vi "FiltJump.vi"(9 "LowLim":sgl, 10 "HighLim":sgl, 11 "Path":T2) -> (3 "PathOut":T2)   [LabVIEW 2014]
uses:
  TypeDefs/Point2DwSlope.ctl
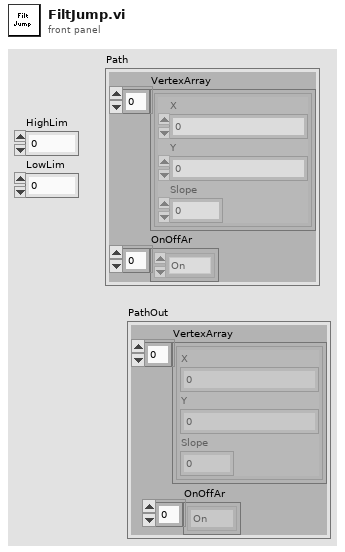
[diagram p1: front panel]
types:
  T1 = typedef "Point2DwSlope.ctl" = cluster{"X":sgl, "Y":sgl, "Slope":dbl}
  T2 = cluster{"VertexArray":T1[], "OnOffAr":enum16{"On", "Off"}[]}
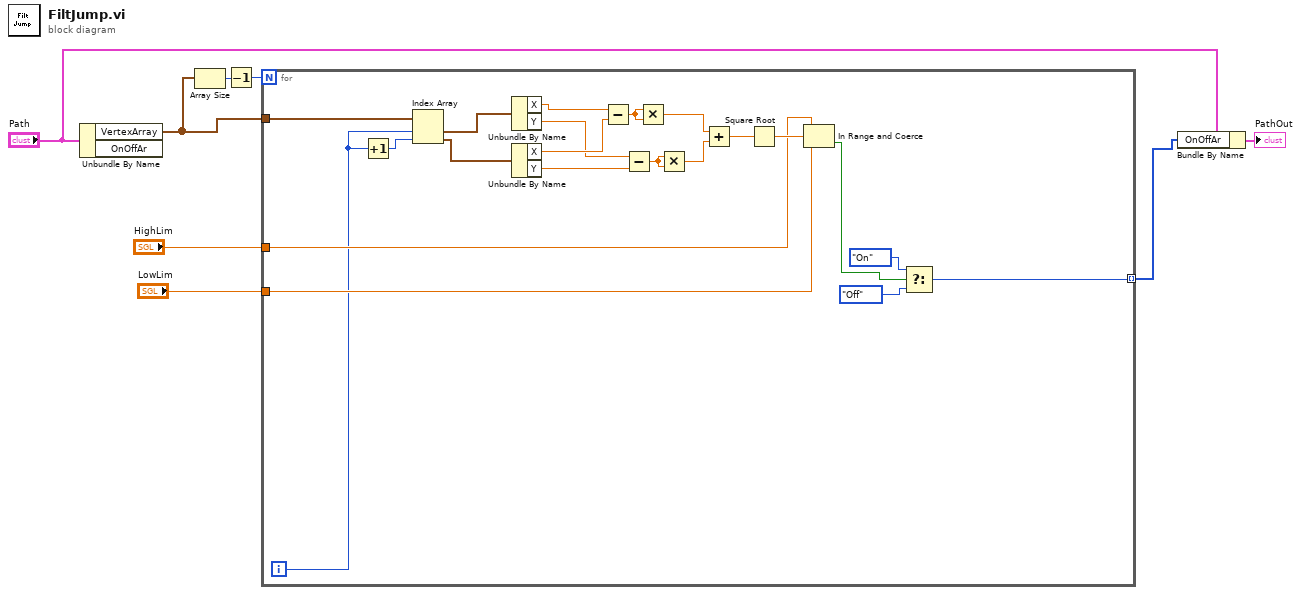
[diagram p0: block diagram]
diagram:
  n1 = Unbundle By Name("Path") -> ("VertexArray"=w8:T1[])  [unwired: 1 out]
  n2 = Array Size(array=w8) -> (size(s)=w7:i32)
  n3 = Decrement(x=w7) -> (x-1=w6:i32)
  n4 = for {
    N: w6 -> [_]
    tunnel: w8 -> [w29]
    tunnel: "HighLim" -> [w15]
    tunnel: "LowLim" -> [w14]
    tunnel: [w9] -> w1 mode=indexing
    i -> [w13]
    n5 = Increment(x=w13) -> (x+1=w28:i32)
    n6 = Index Array(array=w29, index #1=w13, index #2=w28) -> (element #1=w27:T1, element #2=w26:T1)
    n7 = Unbundle By Name(w27) -> ("X"=w25:sgl, "Y"=w23:sgl)
    n8 = Unbundle By Name(w26) -> ("X"=w24:sgl, "Y"=w22:sgl)
    n9 = Subtract(x=w25, y=w24) -> (x-y=w21:sgl)
    n10 = Subtract(x=w23, y=w22) -> (x-y=w20:sgl)
    n11 = Multiply(x=w21, y=w21) -> (x*y=w19:sgl)
    n12 = Multiply(x=w20, y=w20) -> (x*y=w18:sgl)
    n13 = Add(x=w19, y=w18) -> (x+y=w17:sgl)
    n14 = Square Root(x=w17) -> (sqrt(x)=w16:sgl)
    n15 = In Range and Coerce(upper limit=w15, x=w16, lower limit=w14) -> (In Range?=w11:bool)  [unwired: 1 out]
    n16 = Select(t=enum16{"On", "Off"}."On" ("new element/subarray"), s=w11, f=enum16{"On", "Off"}."Off" ("new element/subarray")) -> (s? t:f=w9:enum16{"On", "Off"})
  }
  n17 = Bundle By Name(cluster="Path", "OnOffAr"=w1) -> (→"PathOut":T2)
